vi "set_H2N2remote.vi"(0 "H2N2 Remote":bool) -> ()   [LabVIEW 2011]
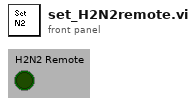
[diagram p1: front panel]
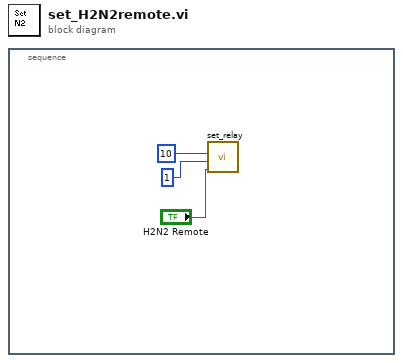
[diagram p0: block diagram]
diagram:
  n1 = stacked-sequence {
    frame #0 {
      n2 = call "set_relay.vi"("Slot"=10, "Relay"=1, "Relay Status"="H2N2 Remote") -> ()  [unwired: 3 out]
    }
  }
